vi "tsp.vi"() -> ()   [LabVIEW 2024]
uses:
  <vilib>/numeric/Random Number (Range) U64.vi
  <vilib>/numeric/Random Number (Range) I64.vi
  <vilib>/numeric/sub_Random U32.vi
panel:
  in  "Array":dbl[](array[numeric])
  out "Waveform Graph":dbl[](graph)
  out "cnt":i32
  out "best_score":dbl
  out "XY Graph 2":cluster{u64[], u64[]}(graph)
  in  "cnt_max":i32
  out "y_pos":u64[](array[numeric])
  out "x_pos":u64[](array[numeric])
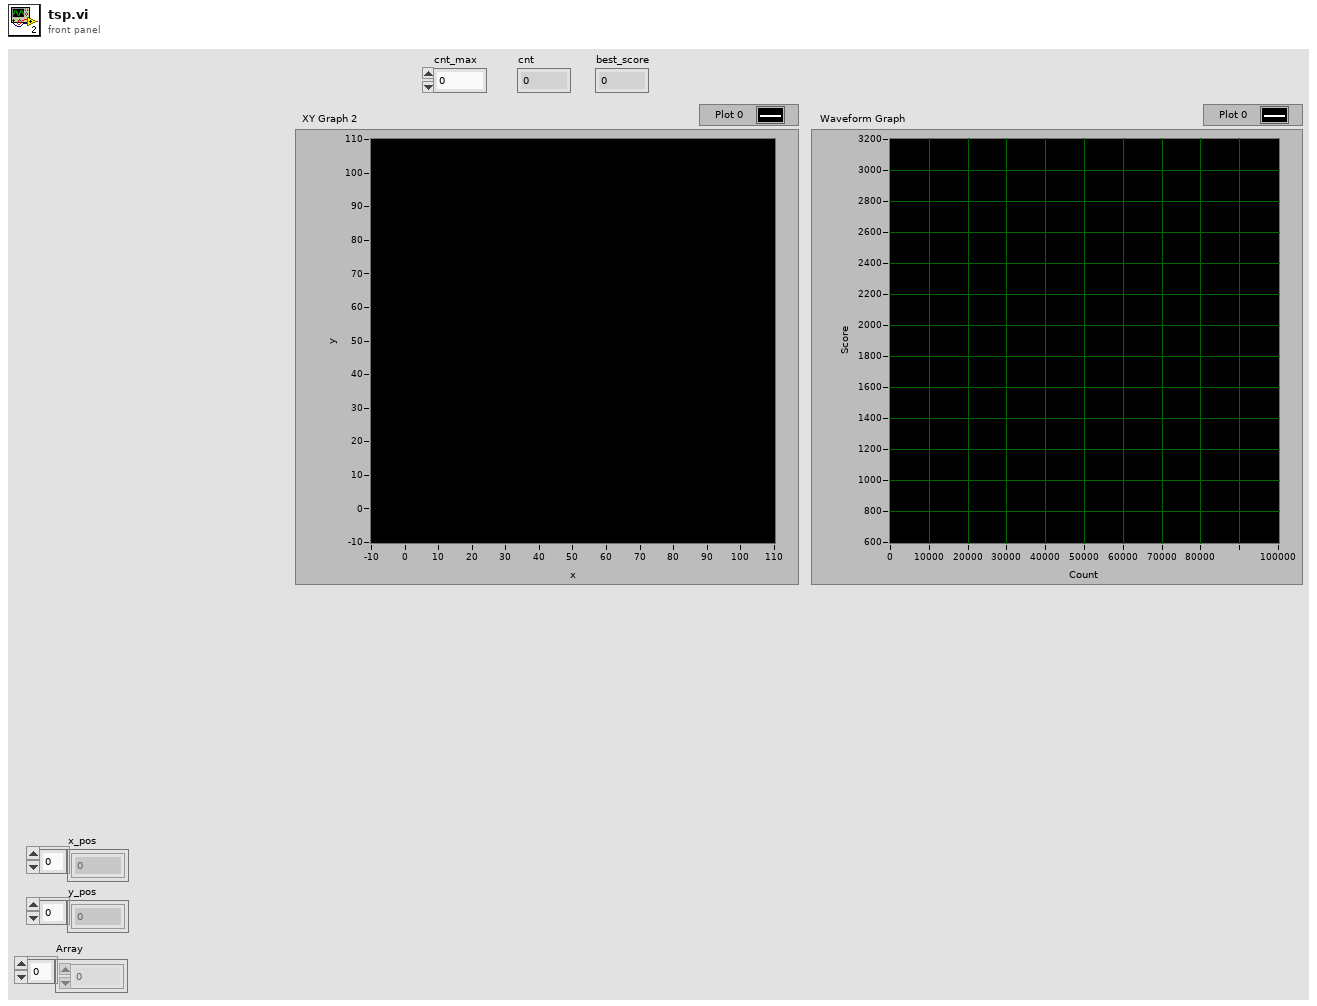
[diagram p1: front panel]
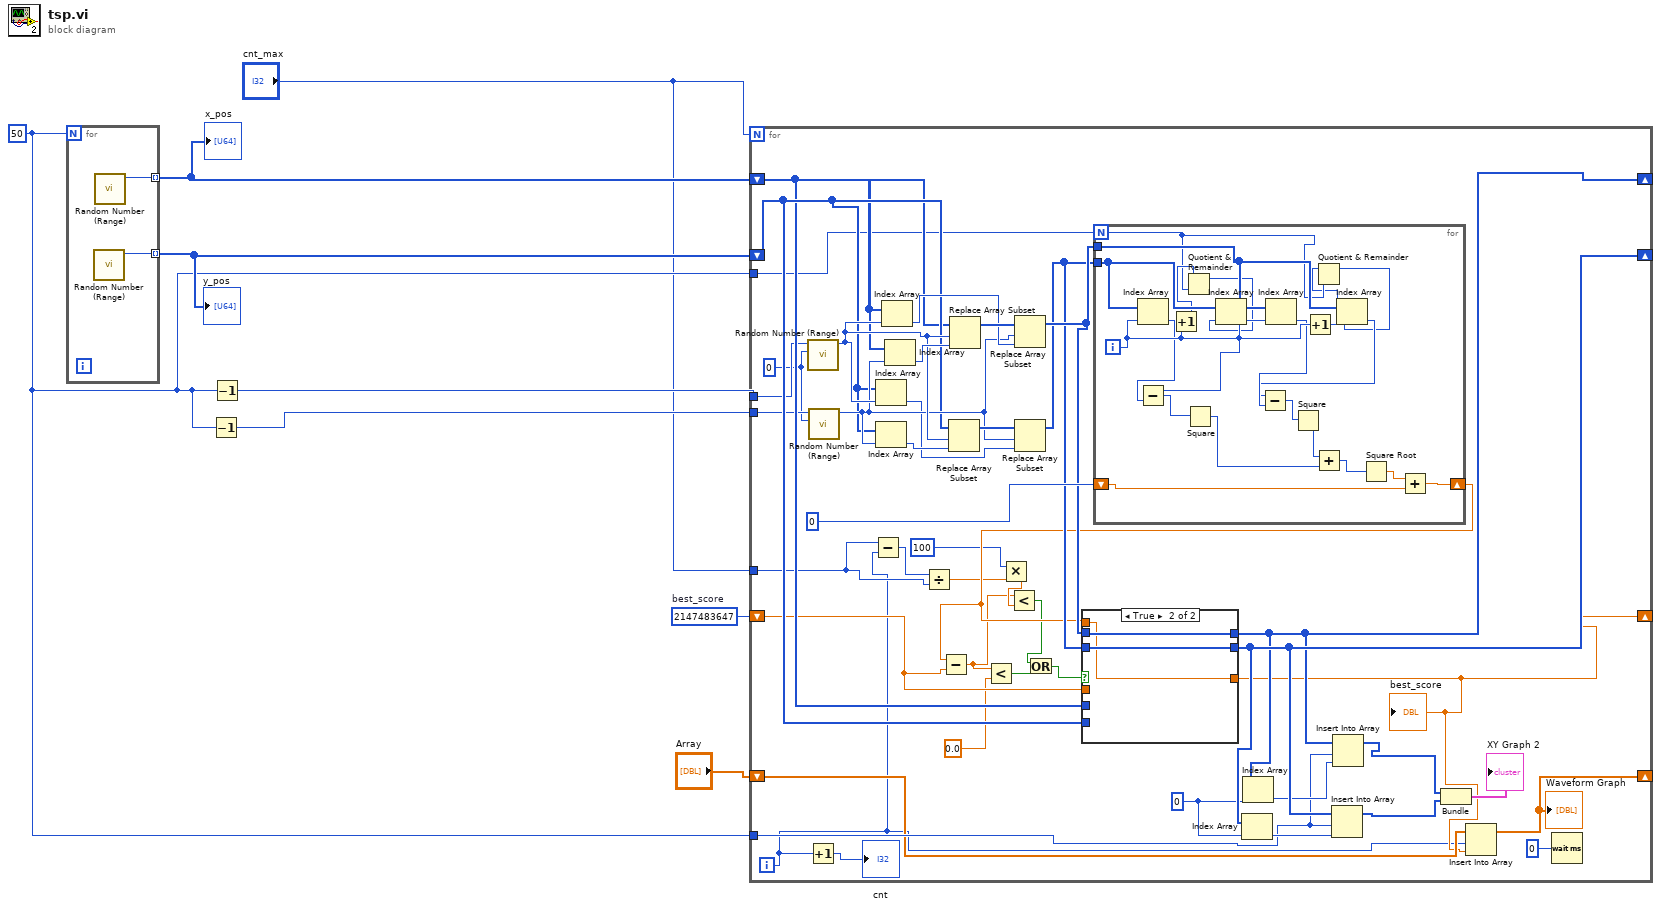
[diagram p0: block diagram]
diagram:
  w6 = 2147483647  # best_score
  w3 = 50
  n1 = for {
    N: w3 -> [_]
    tunnel: [w10] -> w8 mode=indexing
    tunnel: [w9] -> w7 mode=indexing
    n2 = call-poly <vilib>:"Random Number (Range).vi"() -> ("number"=w9:u64)  [unwired: 11 in]
    n3 = call-poly <vilib>:"Random Number (Range).vi"() -> ("number"=w10:u64)  [unwired: 11 in]
  }
  "x_pos" <- w8
  "y_pos" <- w7
  n4 = Decrement(x=w3) -> (x-1=w4:i32)
  n5 = Decrement(x=w3) -> (x-1=w5:i32)
  n6 = for {
    N: "cnt_max" -> [_]
    shift-right: [w14] -> _
    shift-left: w6 -> [w27]
    shift-right: [w31] -> _
    shift-left: w8 -> [w40]
    shift-right: [w34] -> _
    shift-left: w7 -> [w41]
    tunnel: w5 -> [w39]
    tunnel: w4 -> [w38]
    tunnel: w3 -> [w36]
    tunnel: w3 -> [w28]
    tunnel: "cnt_max" -> [w18]
    shift-right: [w12] -> _
    shift-left: "Array" -> [w15]
    i -> [w13]
    w30 = 0
    w37 = i64 0 ("lower bound (-100)")
    n7 = call-poly <vilib>:"Random Number (Range).vi"("lower bound (-100)"=w37, "upper bound (100)"=w39) -> ("number"=w49:i64)  [unwired: 9 in]
    n8 = Increment(x=w13) -> (x+1=→"cnt":i32)
    n9 = call-poly <vilib>:"Random Number (Range).vi"("lower bound (-100)"=w37, "upper bound (100)"=w38) -> ("number"=w46:i64)  [unwired: 9 in]
    n10 = Subtract(x=w18, y=w13) -> (x-y=w17:i32)
    n11 = Index Array(array=w41, index=w49) -> (element=w45:u64)
    n12 = Index Array(array=w41, index=w46) -> (element=w48:u64)
    n13 = Index Array(array=w40, index=w49) -> (element=w50:u64)
    n14 = Index Array(array=w40, index=w46) -> (element=w52:u64)
    n15 = Divide(x=w17, y=w18) -> (x/y=w22:dbl)
    n16 = Replace Array Subset(array=w41, new element=w48, index=w49) -> (w47:u64[])
    n17 = Replace Array Subset(array=w40, new element=w52, index=w49) -> (w51:u64[])
    n18 = Multiply(x=100, y=w22) -> (x*y=w21:dbl)
    n19 = Replace Array Subset(array=w51, new element=w50, index=w46) -> (w43:u64[])
    n20 = Replace Array Subset(array=w47, new element=w45, index=w46) -> (w42:u64[])
    n21 = for {
      N: w36 -> [w62]
      tunnel: w42 -> [w80]
      tunnel: w43 -> [w79]
      shift-right: [w66] -> w26
      shift-left: 0 -> [w67]
      i -> [w78]
      n22 = Index Array(array=w80, index=w78) -> (element=w77:u64)
      n23 = Increment(x=w78) -> (x+1=w63:i32)
      n24 = Quotient & Remainder(x=w63, y=w62) -> (x-y*floor(x/y)=w65:i32)  [unwired: 1 out]
      n25 = Index Array(array=w80, index=w65) -> (element=w76:u64)
      n26 = Subtract(x=w76, y=w77) -> (x-y=w75:u64)
      n27 = Square(x=w75) -> (x^2=w70:u64)
      n28 = Index Array(array=w79, index=w78) -> (element=w74:u64)
      n29 = Increment(x=w78) -> (x+1=w61:i32)
      n30 = Quotient & Remainder(x=w61, y=w62) -> (x-y*floor(x/y)=w64:i32)  [unwired: 1 out]
      n31 = Index Array(array=w79, index=w64) -> (element=w73:u64)
      n32 = Subtract(x=w73, y=w74) -> (x-y=w72:u64)
      n33 = Square(x=w72) -> (x^2=w71:u64)
      n34 = Add(x=w71, y=w70) -> (x+y=w69:u64)
      n35 = Square Root(x=w69) -> (sqrt(x)=w68:dbl)
      n36 = Add(x=w68, y=w67) -> (x+y=w66:dbl)
    }
    n37 = Subtract(x=w26, y=w27) -> (x-y=w20:dbl)
    n38 = Less?(x=w20, y=0.0) -> (x < y?=w24:bool)
    n39 = Less?(x=w20, y=w21) -> (x < y?=w19:bool)
    n40 = Or(x=w19, y=w24) -> (x .or. y?=w23:bool)
    n41 = case shown="True" w23 {
      tunnel: w43 -> [_ w60]
      tunnel: w42 -> [_ w59]
      tunnel: w41 -> [w56 _]
      tunnel: w40 -> [w57 _]
      tunnel: [w57 w60] -> w31
      tunnel: [w56 w59] -> w34
      tunnel: w27 -> [w55 _]
      tunnel: w26 -> [_ w58]
      tunnel: [w55 w58] -> w14
      frame False {
      }
      frame True {
      }
    }
    "best_score" <- w14
    n42 = Index Array(array=w34, index=w30) -> (element=w33:u64)
    n43 = Index Array(array=w31, index=w30) -> (element=w32:u64)
    n44 = Insert Into Array(array=w34, index=w28, new element=w33) -> (w29:u64[])
    n45 = Insert Into Array(array=w31, index=w28, new element=w32) -> (w35:u64[])
    n46 = Bundle(w35, w29) -> (→"XY Graph 2":cluster{u64[], u64[]})  [unwired: 1 in]
    n47 = Insert Into Array(array=w15, index=w13, new element=w14) -> (w12:dbl[])
    "Waveform Graph" <- w12
    n48 = Wait (ms)(milliseconds to wait=u32 0) -> ()  [unwired: 1 out]
  }
